vi "Configure Island Watch.vi"(5 "Island stop notifier":refnum<notifier>, 6 "Frequency Control":refnum<class "Message Enqueuer.lvclass">, 7 "Register":u16, 8 "error in (no error)":errorcluster, 10 "Modbus Handle":refnum<class "Modbus Master.lvclass">, 11 "Island Watch in":refnum<class "Island Watch.lvclass">) -> (0 "error out":errorcluster, 3 "Island Watch out":refnum<class "Island Watch.lvclass">)   [LabVIEW 2015, in "Island Watch Actor.lvlib" / "Island Watch.lvclass"]
uses:
  Island Watch.lvclass
  <vilib>/ActorFramework/Message Enqueuer/Message Enqueuer.lvclass
  <vilib>/Modbus/master/Modbus Master.lvclass
  Island Watch.lvclass/Island Watch.ctl
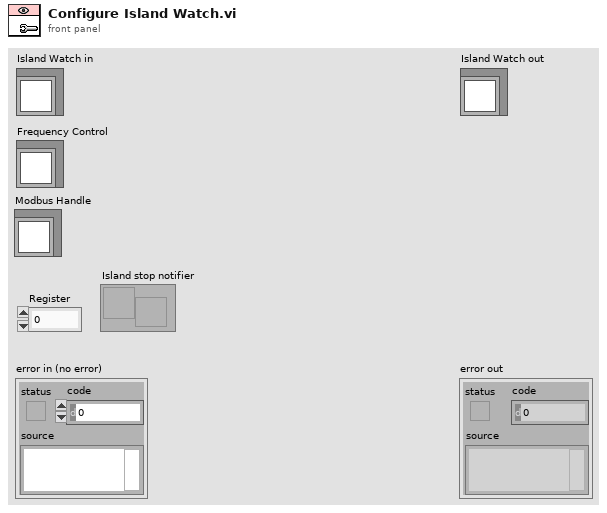
[diagram p1: front panel]
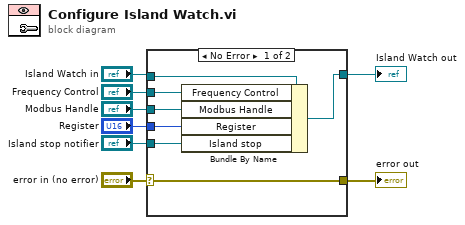
[diagram p0: block diagram]
diagram:
  n1 = case shown="No Error" "error in (no error)" {
    selector: "error in (no error)" -> [w14 w17]
    tunnel: [w14 w17] -> w7
    tunnel: [w13 w16] -> w5
    tunnel: "Island Watch in" -> [w15 w16]
    tunnel: "Frequency Control" -> [w12 _]
    tunnel: "Register" -> [w11 _]
    tunnel: "Modbus Handle" -> [w10 _]
    tunnel: "Island stop notifier" -> [w9 _]
    frame No Error {
      n2 = Bundle By Name(cluster=w15, "Frequency Control"=w12, "Modbus Handle"=w10, "Register"=w11, "Island stop"=w9) -> (w13:refnum<class "Island Watch.lvclass">)
    }
    frame Error {
    }
  }
  "error out" <- w7
  "Island Watch out" <- w5
